vi "Handle Error.vi"(8 "error in (no error)":errorcluster, 11 "Car Wash Controller in":refnum<class "Car Wash Controller.lvclass">) -> (0 "error out":errorcluster, 2 "stop actor?":bool=TRUE, 3 "Car Wash Controller out":refnum<class "Car Wash Controller.lvclass">)   [LabVIEW 2012, in "Car Wash Controller.lvlib" / "Car Wash Controller.lvclass"]
doc: "(<B>Filename</B>: Actor Framework.lvlib:Actor.lvclass:Handle Error.vi)\n\nDefines how the actor handles an error that occurred while processing a message.\n\nBy default, this method does nothing except stop the actor. This method also treats error code 43 (coming from <B>error in</B>) as a sign that the actor shut down normally. In this situation, the Handle Error method does not return the error on <B>error out</B>, meaning the actor's caller will not receive it. All other error codes will be returned on <B>error out</B>.\n\nA descendant class may override this method to change this behavior."
uses:
  Car Wash Controller.lvclass
  <vilib>/ActorFramework/Actor/Actor.lvclass
  Car Wash Controller State.ctl
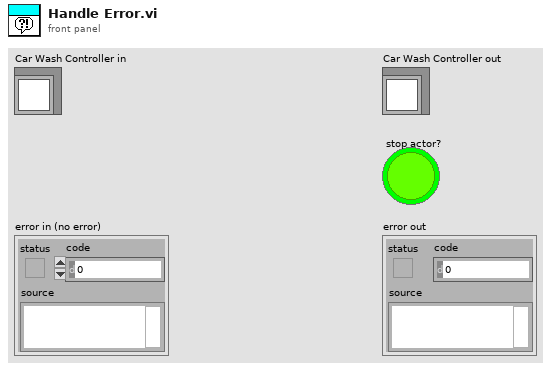
[diagram p1: front panel]
types:
  T1 = typedef "Car Wash Controller.lvlib/Car Wash Controller.lvclass/Car Wash Controller State.ctl" = enum16{"Initial State", "Wait For Start State", "Start State", "Wait For Vehicle Position State", "Wash Step Execution State", "Wash Step / Cycle Completion State", "Wash Exit State", "Wash Abort / Terminate State"}
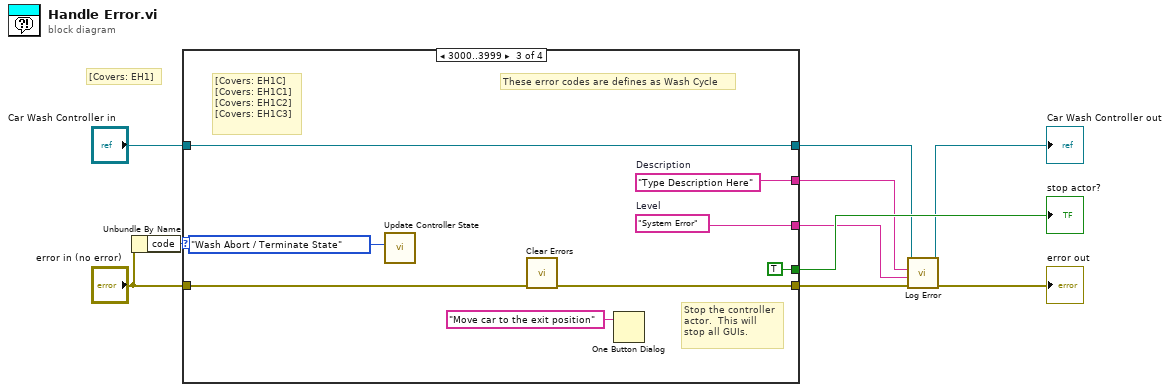
[diagram p0: block diagram]
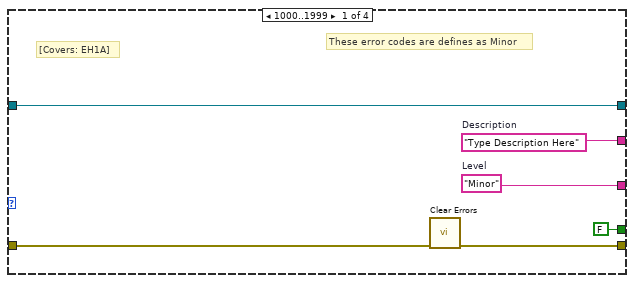
[diagram p2: hidden frame]
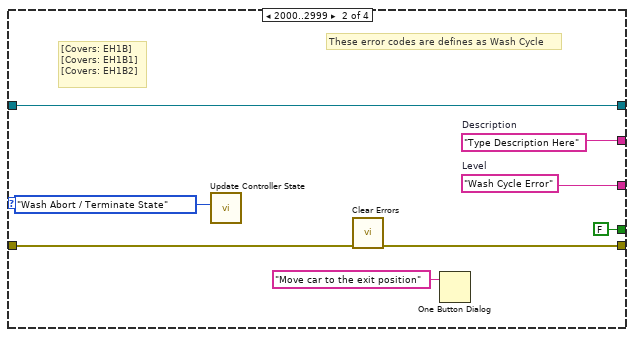
[diagram p3: hidden frame]
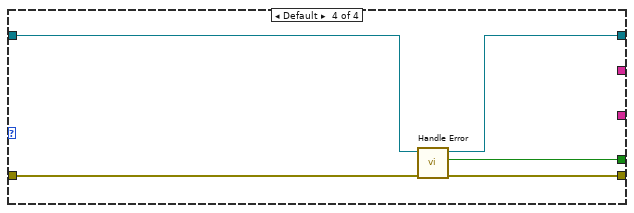
[diagram p4: hidden frame]
diagram:
  # "[Covers: EH1]"
  n1 = Unbundle By Name("error in (no error)") -> ("code"=w6:i32)
  n2 = case shown="3000..3999" w6 {
    tunnel: [w14 w17 w25 w37] -> w10
    tunnel: [FALSE ("stop actor?") FALSE ("stop actor?") TRUE ("stop actor?") w36] -> w9
    tunnel: [w16 w24 w32 w35] -> w3
    tunnel: "error in (no error)" -> [w15 w18 w26 w34]
    tunnel: "Car Wash Controller in" -> [w16 w24 w32 w33]
    tunnel: [w12 w22 w30 _] -> w2
    tunnel: [w11 w21 w29 _] -> w1
    frame 1000..1999 {
      w11 = "Minor"  # Level
      w12 = "Type Description Here"  # Description
      # "[Covers: EH1A]"
      # "These error codes are defines as Minor"
      n3 = call <vilib>:"Clear Errors.vi"("error in (no error)"=w15) -> ("error out"=w14:errorcluster)  [unwired: 5 in, 1 out]
    }
    frame 2000..2999 {
      w21 = "Wash Cycle Error"  # Level
      w22 = "Type Description Here"  # Description
      # "[Covers: EH1B]\n[Covers: EH1B1]\n[Covers: EH1B2]"
      # "These error codes are defines as Wash Cycle"
      n4 = call "Update Controller State.vi"("Car Wash Controller State"=Car_Wash_Controller_State."Wash Abort / Terminate State") -> ()  [unwired: 9 in, 2 out]
      n5 = call <vilib>:"Clear Errors.vi"("error in (no error)"=w18) -> ("error out"=w17:errorcluster)  [unwired: 5 in, 1 out]
      n6 = One Button Dialog(message="Move car to the exit position") -> ()  [unwired: 1 in, 1 out]
    }
    frame 3000..3999 {
      w29 = "System Error"  # Level
      w30 = "Type Description Here"  # Description
      # "[Covers: EH1C]\n[Covers: EH1C1]\n[Covers: EH1C2]\n[Covers: EH1C3]"
      # "Stop the controller\nactor.  This will\nstop all GUIs."
      # "These error codes are defines as Wash Cycle"
      n7 = call "Update Controller State.vi"("Car Wash Controller State"=Car_Wash_Controller_State."Wash Abort / Terminate State") -> ()  [unwired: 9 in, 2 out]
      n8 = call <vilib>:"Clear Errors.vi"("error in (no error)"=w26) -> ("error out"=w25:errorcluster)  [unwired: 5 in, 1 out]
      n9 = One Button Dialog(message="Move car to the exit position") -> ()  [unwired: 1 in, 1 out]
    }
    frame Default {
      n10 = call-parent "Handle Error.vi"("error in (no error)"=w34, "Actor in"=w33) -> ("error out"=w37:errorcluster, "stop actor?"=w36:bool, "Actor out"=w35:refnum<class "Car Wash Controller.lvclass">)  [unwired: 7 in]
    }
  }
  "stop actor?" <- w9
  n11 = call "Log Error.vi"("error in (no error)"=w10, "Level"=w1, "Description"=w2, "Car Wash Controller in"=w3) -> ("error out"=→"error out":errorcluster, "Car Wash Controller out"=→"Car Wash Controller out":refnum<class "Car Wash Controller.lvclass">)  [unwired: 6 in]
